vi "pp2_DAQplayAudio.vi"(0 "Daq config In":T1={"Sound AO"="Dev2/ao0", "Shock intesity AO"="Dev1/ao1", "Code_LED DO"="Dev1/port1:2", "Switches DI"="Dev1/port0/line0:1", "Webcam"="cam0", "Sound AO task"="", "Sound card task"=0, "Shock intensity AO task"="", "Code_LED DO task"="", "Switch DI task"="", "AO <=> Sound card"=FALSE, "Sound card"=0, "sample rate"=8000.0, "Variable shock"=FALSE, "Webcam on"=FALSE, "Tone gate PFI"="/Dev1/PFI1", "Waveform memo"={"t0"=timestamp(0 s since 1904-01-01), "dt"=1.0, "Y"=[]}} {"sample rate" min=8000.0; "Sound card task" format="%.0x"}, 5 "Tone countdown (ms) In":i64, 7 "Tone repeat memo":i64, 11 "error in (no error)":errorcluster) -> (4 "Daq config Out":T1={"Sound AO"="Dev2/ao0", "Shock intesity AO"="Dev1/ao1", "Code_LED DO"="Dev1/port1:2", "Switches DI"="Dev1/port0/line0:1", "Webcam"="cam0", "Sound AO task"="", "Sound card task"=0, "Shock intensity AO task"="", "Code_LED DO task"="", "Switch DI task"="", "AO <=> Sound card"=FALSE, "Sound card"=0, "sample rate"=8000.0, "Variable shock"=FALSE, "Webcam on"=FALSE, "Tone gate PFI"="/Dev1/PFI1", "Waveform memo"={"t0"=timestamp(0 s since 1904-01-01), "dt"=1.0, "Y"=[]}} {"sample rate" min=8000.0; "Sound card task" format="%.0x"}, 6 "Tone countdown (ms) Out":i64, 15 "error out":errorcluster)   [LabVIEW 2013]
uses:
  pp2_CTL_DaqConfig.ctl
  <vilib>/userdefined/High Color/IMAQdx.ctl
  <vilib>/sound2/lvsound2.llb/Sound Output Task ID.ctl
  <vilib>/sound2/lvsound2.llb/Sound Output Write (DBL Single).vi
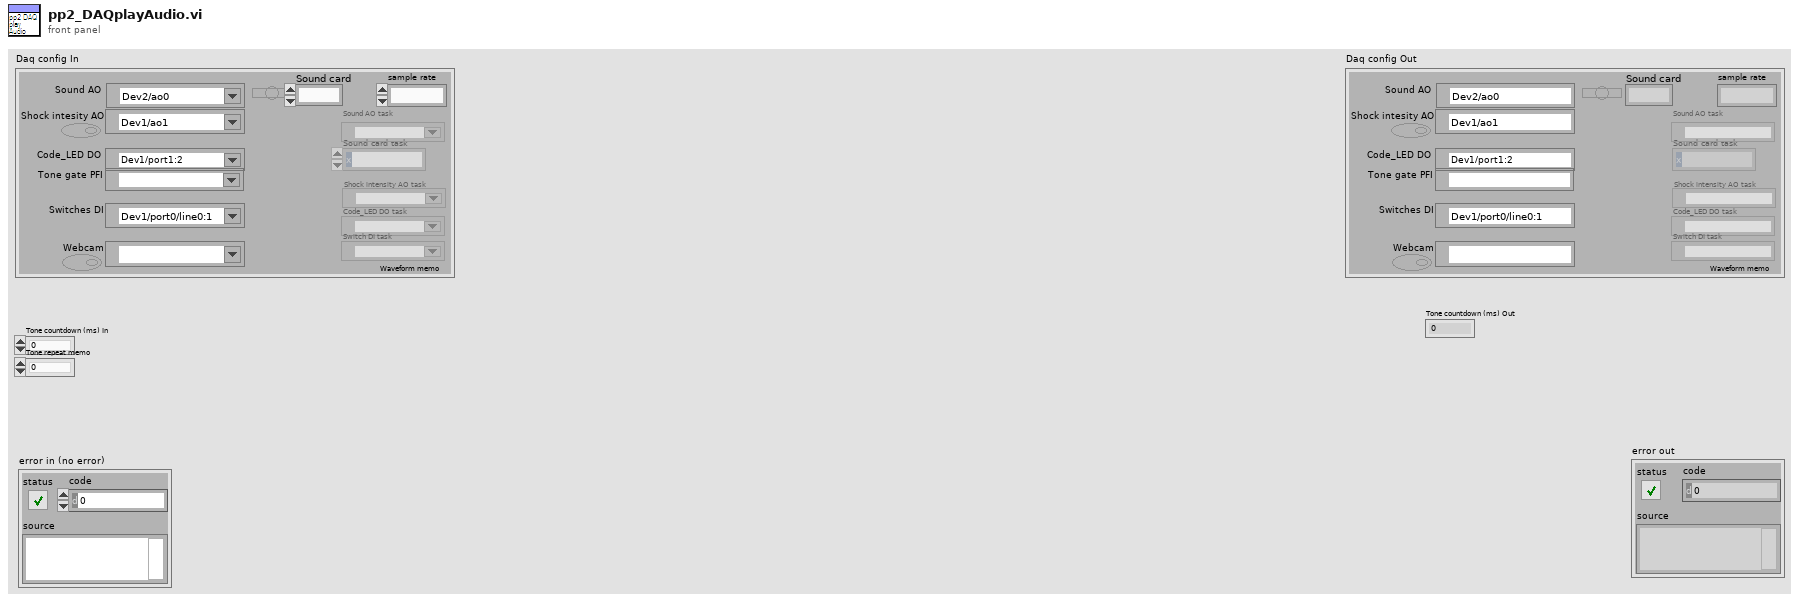
[diagram p1: front panel]
types:
  T1 = typedef "pp2_CTL_DaqConfig.ctl" = cluster{"Sound AO":tag, "Shock intesity AO":tag, "Code_LED DO":tag, "Switches DI":tag, "Webcam":T2, "Sound AO task":refnum<k21>, "Sound card task":T3, "Shock intensity AO task":refnum<k21>, "Code_LED DO task":refnum<k21>, "Switch DI task":refnum<k21>, "AO <=> Sound card":bool, "Sound card":u32, "sample rate":dbl, "Variable shock":bool, "Webcam on":bool, "Tone gate PFI":tag, "Waveform memo":waveform(dbl)}
  T2 = typedef "IMAQdx.ctl" = refnum<k21>
  T3 = typedef "Sound Output Task ID.ctl" = u32
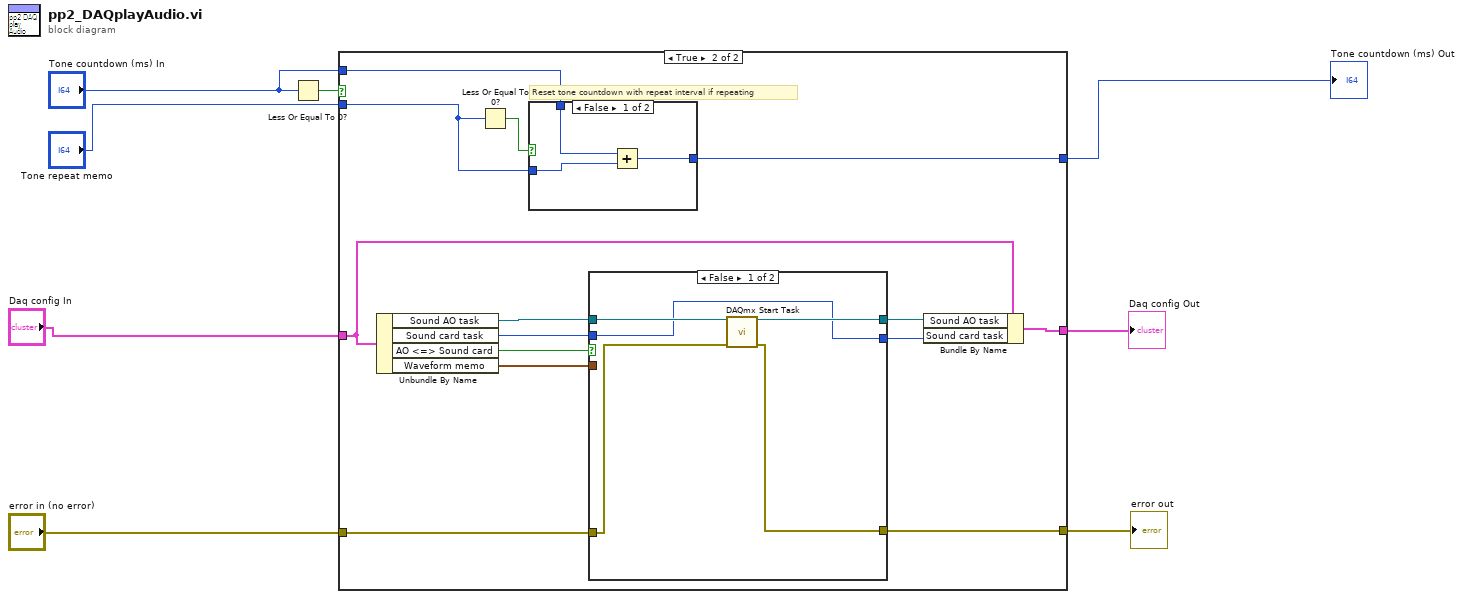
[diagram p0: block diagram]
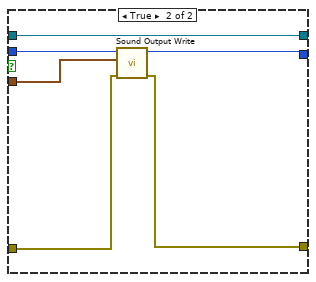
[diagram p3: hidden frame]
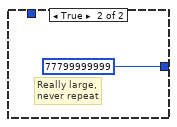
[diagram p4: hidden frame]
diagram:
  n1 = Less Or Equal To 0?(x="Tone countdown (ms) In") -> (x <= 0?=w8:bool)
  n2 = case shown="True" w8 {
    tunnel: [w9 w24] -> w2
    tunnel: "Tone repeat memo" -> [_ w23]
    tunnel: "Daq config In" -> [w11 w19]
    tunnel: [w11 w18] -> w6
    tunnel: "error in (no error)" -> [w10 w15]
    tunnel: [w10 w14] -> w4
    tunnel: "Tone countdown (ms) In" -> [w9 w12]
    frame False {
      # "Don't touch tone countdown (i.e. don't reset) if > 0"
    }
    frame True {
      # "Reset tone countdown with repeat interval if repeating"
      n3 = Unbundle By Name(w19) -> ("Sound AO task"=w21:refnum<k21>, "Sound card task"=w20:T3, "AO <=> Sound card"=w22:bool, "Waveform memo"=w13:waveform(dbl))
      n4 = Less Or Equal To 0?(x=w23) -> (x <= 0?=w25:bool)
      n5 = case shown="False" w25 {
        tunnel: [w39 i64 77799999999 ("Tone countdown (ms)")] -> w24
        tunnel: w23 -> [w38 _]
        tunnel: w12 -> [w37 _]
        frame False {
          n6 = Add(x=w37, y=w38) -> (x+y=w39:i64)
        }
        frame True {
          # "Really large,\nnever repeat"
        }
      }
      n7 = case shown="False" w22 {
        tunnel: w21 -> [w30 w34]
        tunnel: w20 -> [w28 w36]
        tunnel: [w29 w34] -> w17
        tunnel: [w28 w35] -> w16
        tunnel: w15 -> [w27 w32]
        tunnel: [w26 w31] -> w14
        tunnel: w13 -> [_ w33]
        frame False {
          n8 = call <vilib>:"DAQmx Start Task.vi"("task/channels in"=w30, "error in"=w27) -> ("task out"=w29:refnum<k21>, "error out"=w26:errorcluster)  [unwired: 12 in]
        }
        frame True {
          n9 = call-poly <vilib>:"Sound Output Write.vi"("error in (no error)"=w32, "data"=w33, "task ID"=w36) -> ("error out"=w31:errorcluster, "task ID out"=w35:T3)  [unwired: 7 in]
        }
      }
      n10 = Bundle By Name(cluster=w19, "Sound AO task"=w17, "Sound card task"=w16) -> (w18:T1)
    }
  }
  "Daq config Out" <- w6
  "error out" <- w4
  "Tone countdown (ms) Out" <- w2
